vi "deceltobun.vi"() -> ()   [LabVIEW 2014, in "Panels.lvlib"]
uses:
  Panels.lvlib
  CSlibraries-extern/DimLVEvent/DimIndicators/DimIndicators.lvlib
  CSlibraries/UtilityLib/UtilityLib.lvlib
  CS_Core/CSSystem/CoreLib/CoreLib.lvlib
  CSlibraries/UtilityLib/UtilityLib.valueStatus.ctl
  CSlibraries-extern/DimLVEvent/LVDimInterface/LVDimInterface.lvlib
  Instance           1 18Saved   deceltobun .vi
  Instance           2 18Saved   deceltobun .vi
  CSlibraries-extern/DimLVEvent/DimIndicators/DimIndicators.numericArrayType.ctl
  CSlibraries-extern/DimLVEvent/DimIndicators/DimIndicators.anyType.ctl
  CSlibraries-extern/DimLVEvent/DimIndicators/DimIndicators.numericType.ctl
panel:
  out "DIM Error":bool
  in  "SetFileLocation_Data":T1={"data"="NOLINK", "no link"=TRUE, "quality"=-1, "timeStamp"=0.0}
  in  "Q90PlanDefY":bool
  in  "ISDefY":bool
  in  "Q90PlanLens":bool
  in  "BOB3DefY":bool
  in  "BOB3DefX":bool
  in  "BOB2Q90Lens":bool
  in  "Q90DefMain":bool
  in  "Q90BOB3Lens":bool
  in  "ISDefX":bool
  in  "Q90CylLens":bool
  in  "BOB2DefX":bool
  in  "BOB2DefY":bool
  in  "DecelLens":bool
  in  "Decel":bool
  in  "PreBunLens":bool
  in  "Q90DefMain_MonData":T2={"data"=inf, "no link"=FALSE, "quality"=1, "timeStamp"=3265900746.554}
  in  "Q90BOB3Lens_MonData":T2={"data"=inf, "no link"=FALSE, "quality"=1, "timeStamp"=3265900746.538}
  in  "Q90PlanLens_MonData":T2={"data"=inf, "no link"=FALSE, "quality"=1, "timeStamp"=3265900746.522}
  in  "BOB3DefX_MonData":T2={"data"=inf, "no link"=FALSE, "quality"=1, "timeStamp"=3265900746.554}
  in  "Decel_MonData":T2={"data"=inf, "no link"=FALSE, "quality"=1, "timeStamp"=3265900746.538}
  in  "DecelLens_MonData":T2={"data"=inf, "no link"=FALSE, "quality"=1, "timeStamp"=3265900746.569}
  in  "BOB2Q90Lens_MonData":T2={"data"=inf, "no link"=FALSE, "quality"=1, "timeStamp"=3265900746.554}
  in  "ISDefX_MonData":T2={"data"=inf, "no link"=FALSE, "quality"=1, "timeStamp"=3265900746.538}
  in  "BOB2DefX_MonData":T2={"data"=inf, "no link"=FALSE, "quality"=1, "timeStamp"=3265900746.569}
  in  "BOB3DefY_MonData":T2={"data"=inf, "no link"=FALSE, "quality"=1, "timeStamp"=3265900746.569}
  in  "Q90DefCorr1_MonData":T2={"data"=inf, "no link"=FALSE, "quality"=1, "timeStamp"=3265900746.538}
  in  "Q90DefCorr2_MonData":T2={"data"=inf, "no link"=FALSE, "quality"=1, "timeStamp"=3265900746.585}
  in  "Q90PlanDefY_MonData":T2={"data"=inf, "no link"=FALSE, "quality"=1, "timeStamp"=3265900746.538}
  in  "Q90DefMain1_MonData":T2={"data"=inf, "no link"=FALSE, "quality"=1, "timeStamp"=3265900746.554}
  in  "ISDefY_MonData":T2={"data"=inf, "no link"=FALSE, "quality"=1, "timeStamp"=3265900746.522}
  in  "PreBunLens_MonData":T2={"data"=inf, "no link"=FALSE, "quality"=1, "timeStamp"=3265900746.538}
  in  "BOB2DefY_MonData":T2={"data"=inf, "no link"=FALSE, "quality"=1, "timeStamp"=3265900746.6}
  in  "Q90CylLens_MonData":T2={"data"=inf, "no link"=FALSE, "quality"=1, "timeStamp"=3265900746.585}
  in  "Q90DefMain2_MonData":T2={"data"=inf, "no link"=FALSE, "quality"=1, "timeStamp"=3265900746.569}
  in  "Q90DefMain_SetValueInfoData":T3={"data"=[-400.0, 400.0, 3.0], "no link"=FALSE, "quality"=0, "timeStamp"=3265900746.554}
  in  "Q90DefMain_SetData":T3={"data"=[0.0, 0.0, 0.0, 0.0], "no link"=FALSE, "quality"=1, "timeStamp"=3265900745.1}
  out "Q90DefMain_Mon":dbl=inf format="%.4f"
  in  "Decel_SetValueInfoData":T3={"data"=[-404.0, 401.8, 3.0], "no link"=FALSE, "quality"=0, "timeStamp"=3265900746.569}
  in  "Decel_SetData":T3={"data"=[0.0, 0.0, 0.0, 0.0], "no link"=FALSE, "quality"=1, "timeStamp"=3265900745.053}
  out "BOB3DefX_Mon":dbl=inf format="%.4f"
  in  "PreBunLens_SetData":T3={"data"=[0.0, 0.0, 0.0, 0.0], "no link"=FALSE, "quality"=1, "timeStamp"=3265900745.053}
  in  "BOB3DefY_SetValueInfoData":T3={"data"=[-400.0, 400.0, 3.0], "no link"=FALSE, "quality"=0, "timeStamp"=3265900746.554}
  in  "BOB3DefX_SetValueInfoData":T3={"data"=[-400.0, 400.0, 3.0], "no link"=FALSE, "quality"=0, "timeStamp"=3265900746.538}
  in  "Q90BOB3Lens_SetValueInfoData":T3={"data"=[-400.0, 400.0, 3.0], "no link"=FALSE, "quality"=0, "timeStamp"=3265900746.522}
  in  "ISDefY_SetValueInfoData":T3={"data"=[-118.7, 118.8, 3.0], "no link"=FALSE, "quality"=0, "timeStamp"=3265900746.569}
  in  "Q90PlanDefY_SetValueInfoData":T3={"data"=[-120.9, 120.5, 3.0], "no link"=FALSE, "quality"=0, "timeStamp"=3265900746.585}
  in  "Q90PlanLens_SetValueInfoData":T3={"data"=[-120.8, 120.3, 3.0], "no link"=FALSE, "quality"=0, "timeStamp"=3265900746.569}
  in  "BOB3DefY_SetData":T3={"data"=[0.0, 0.0, 0.0, 0.0], "no link"=FALSE, "quality"=1, "timeStamp"=3265900745.1}
  in  "BOB3DefX_SetData":T3={"data"=[0.0, 0.0, 0.0, 0.0], "no link"=FALSE, "quality"=1, "timeStamp"=3265900745.085}
  in  "Q90BOB3Lens_SetData":T3={"data"=[0.0, 0.0, 0.0, 0.0], "no link"=FALSE, "quality"=1, "timeStamp"=3265900745.069}
  in  "ISDefY_SetData":T3={"data"=[0.0, 0.0, 0.0, 0.0], "no link"=FALSE, "quality"=1, "timeStamp"=3265900745.069}
  in  "Q90PlanDefY_SetData":T3={"data"=[0.0, 0.0, 0.0, 0.0], "no link"=FALSE, "quality"=1, "timeStamp"=3265900745.069}
  out "Q90PlanLens_Mon":dbl=inf format="%.4f"
  out "Q90BOB3Lens_Mon":dbl=inf format="%.4f"
  out "BOB3DefY_Mon":dbl=inf format="%.4f"
  out "Q90DefMain1_Mon":dbl=inf format="%.4f"
  out "Q90DefCorr2_Mon":dbl=inf format="%.4f"
  out "Q90DefCorr1_Mon":dbl=inf format="%.4f"
  out "Q90PlanDefY_Mon":dbl=inf format="%.4f"
  in  "Q90PlanLens_SetData":T3={"data"=[0.0, 0.0, 0.0, 0.0], "no link"=FALSE, "quality"=1, "timeStamp"=3265900745.069}
  out "DecelLens_Mon":dbl=inf format="%.4f"
  out "Decel_Mon":dbl=inf format="%.4f"
  out "i ref out":refnum<vi>
  in  "Last Loaded File_Data":T1={"data"="NOLINK", "no link"=TRUE, "quality"=-1, "timeStamp"=0.0}
  out "FileUpToDate":bool=TRUE caption="Parameter Changed"
  in  "Close All Panels":bool
  in  "DecelLens_SetValueInfoData":T3={"data"=[-401.3, 400.4, 3.0], "no link"=FALSE, "quality"=0, "timeStamp"=3265900746.554}
  in  "BOB2Q90Lens_SetValueInfoData":T3={"data"=[-404.3, 403.0, 3.0], "no link"=FALSE, "quality"=0, "timeStamp"=3265900746.538}
  in  "BOB2DefX_SetValueInfoData":T3={"data"=[-400.3, 399.3, 3.0], "no link"=FALSE, "quality"=0, "timeStamp"=3265900746.569}
  in  "BOB2DefY_SetValueInfoData":T3={"data"=[0.0, 3000.0, -1.0], "no link"=FALSE, "quality"=0, "timeStamp"=3265900746.554}
  in  "Q90CylLens_SetValueInfoData":T3={"data"=[0.0, 1500.0, -1.0], "no link"=FALSE, "quality"=0, "timeStamp"=3265900746.554}
  in  "ISDefX_SetValueInfoData":T3={"data"=[0.0, 1000.0, -1.0], "no link"=FALSE, "quality"=0, "timeStamp"=3265900746.538}
  in  "PreBunLens_SetValueInfoData":T3={"data"=[-404.0, 401.8, 3.0], "no link"=FALSE, "quality"=0, "timeStamp"=3265900746.569}
  in  "ISDefX_SetData":T3={"data"=[0.0, 0.0, 0.0, 0.0], "no link"=FALSE, "quality"=1, "timeStamp"=3265900745.069}
  in  "Q90CylLens_SetData":T3={"data"=[0.0, 0.0, 0.0, 0.0], "no link"=FALSE, "quality"=1, "timeStamp"=3265900745.053}
  in  "BOB2DefY_SetData":T3={"data"=[0.0, 0.0, 0.0, 0.0], "no link"=FALSE, "quality"=1, "timeStamp"=3265900745.085}
  in  "BOB2DefX_SetData":T3={"data"=[0.0, 0.0, 0.0, 0.0], "no link"=FALSE, "quality"=1, "timeStamp"=3265900745.085}
  in  "BOB2Q90Lens_SetData":T3={"data"=[0.0, 0.0, 0.0, 0.0], "no link"=FALSE, "quality"=1, "timeStamp"=3265900745.085}
  in  "DecelLens_SetData":T3={"data"=[0.0, 0.0, 0.0, 0.0], "no link"=FALSE, "quality"=1, "timeStamp"=3265900745.053}
  out "Last Loaded File":string
  in  "SetFileLocation":path=path "\\\\Projects\\proj1/lebit/Data Exchange/data/bob1tobunControl"
  out "ISDefY_Mon":dbl=inf format="%.4f"
  out "Q90CylLens_Mon":dbl=inf format="%.4f"
  out "PreBunLens_Mon":dbl=inf format="%.4f"
  out "BOB2DefY_Mon":dbl=inf format="%.4f"
  out "Q90DefMain2_Mon":dbl=inf format="%.4f"
  out "BOB2DefX_Mon":dbl=inf format="%.4f"
  out "ISDefX_Mon":dbl=inf format="%.4f"
  out "BOB2Q90Lens_Mon":dbl=inf format="%.4f"
  # "Parameter changed, data file is no longer up-to-date."
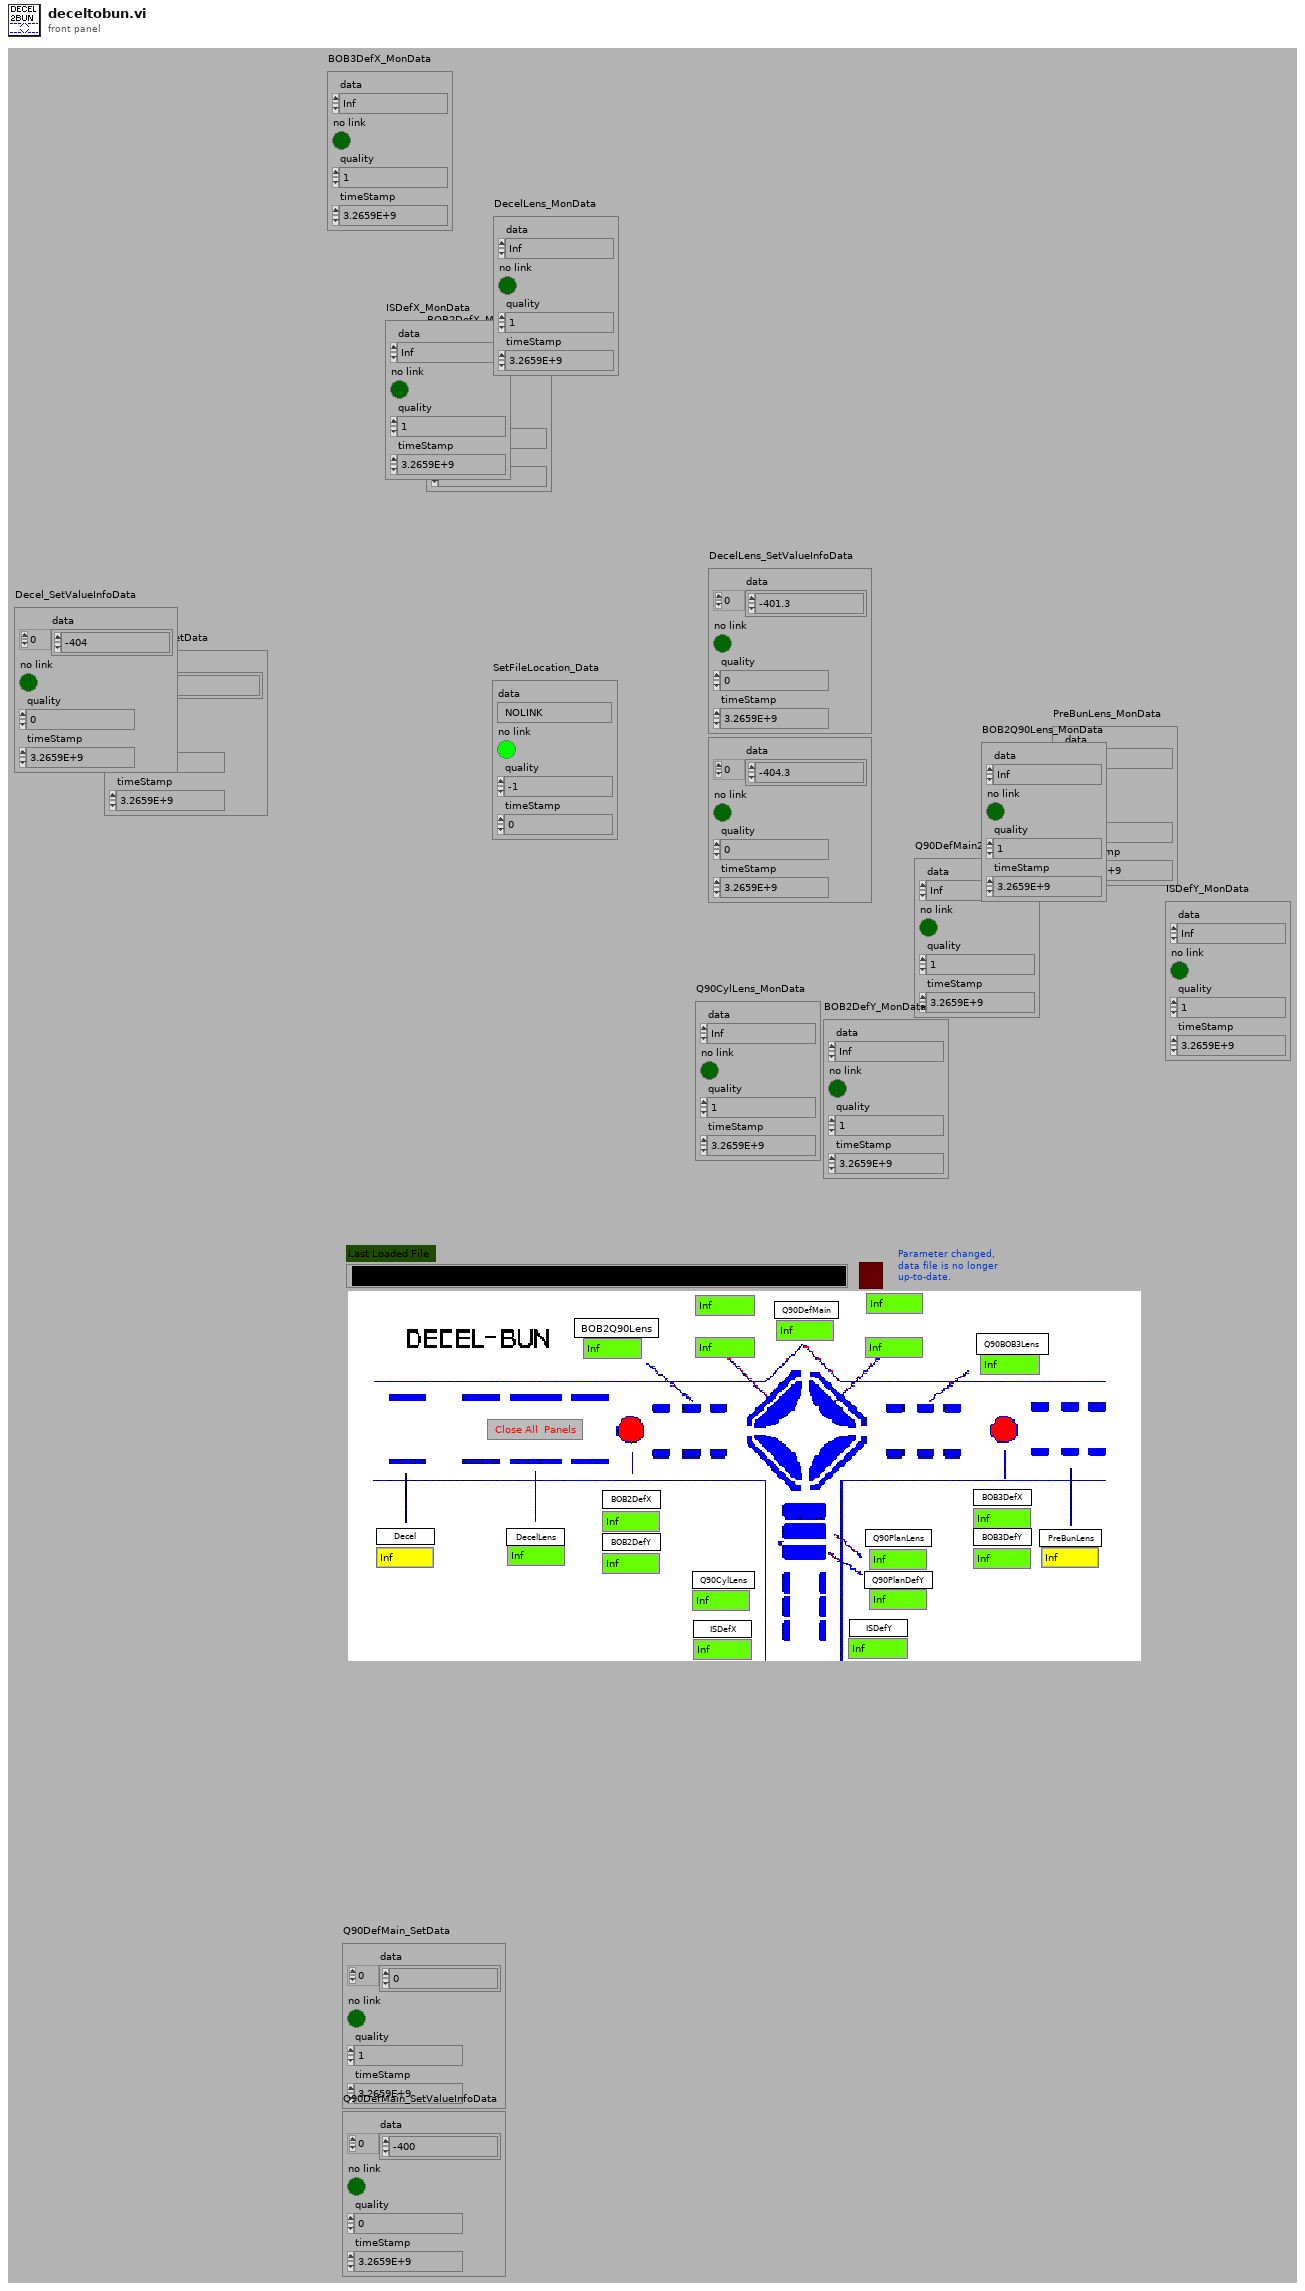
[diagram p1: front panel]
types:
  T1 = typedef "DimIndicators.lvlib/DimIndicators.anyType.ctl" = cluster{"data":string, "no link":bool, "quality":i32, "timeStamp":dbl}
  T2 = typedef "DimIndicators.lvlib/DimIndicators.numericType.ctl" = cluster{"data":dbl, "no link":bool, "quality":i32, "timeStamp":dbl}
  T3 = typedef "DimIndicators.lvlib/DimIndicators.numericArrayType.ctl" = cluster{"data":dbl[], "no link":bool, "quality":i32, "timeStamp":dbl}
  T4 = typedef "UtilityLib.lvlib/UtilityLib.valueStatus.ctl" = enum16{"no info available", "stand by/off", "on", "warning", "alarm/malfunction", "not implemented", "user action required", "important information", "system default", "control default", "indicator default", "button default"}
  T5 = cluster{"data":string, "no link":bool, "quality":i32, "timeStamp":dbl}
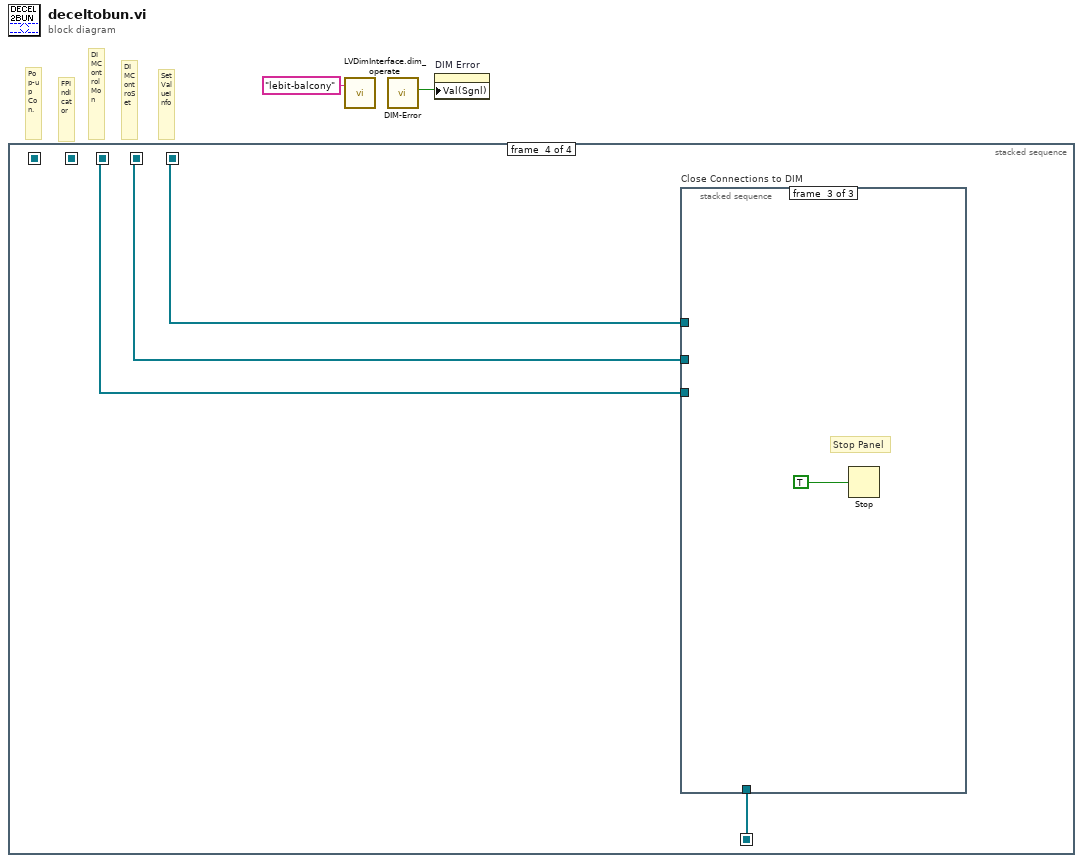
[diagram p0: block diagram]
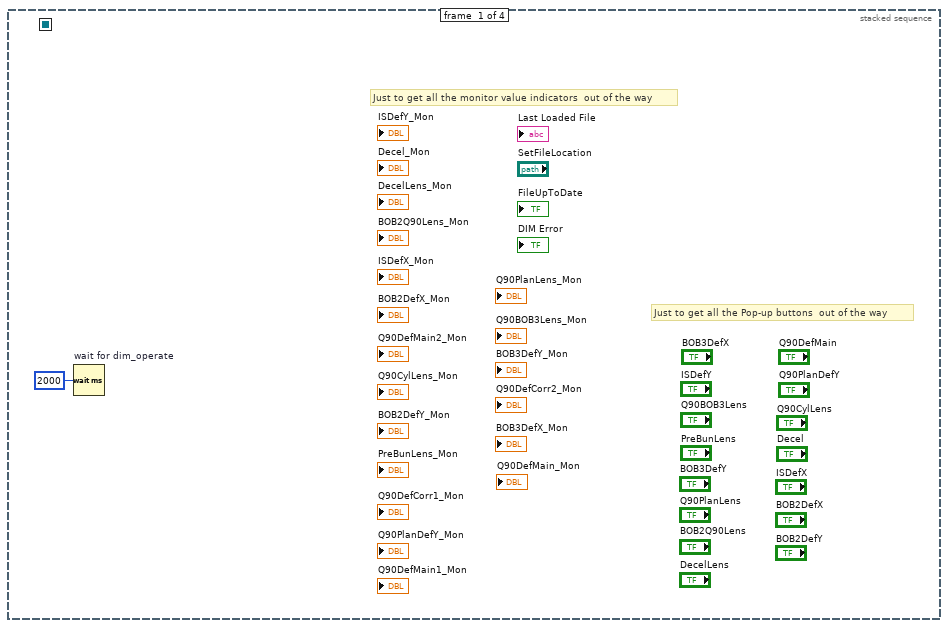
[diagram p2: hidden frame]
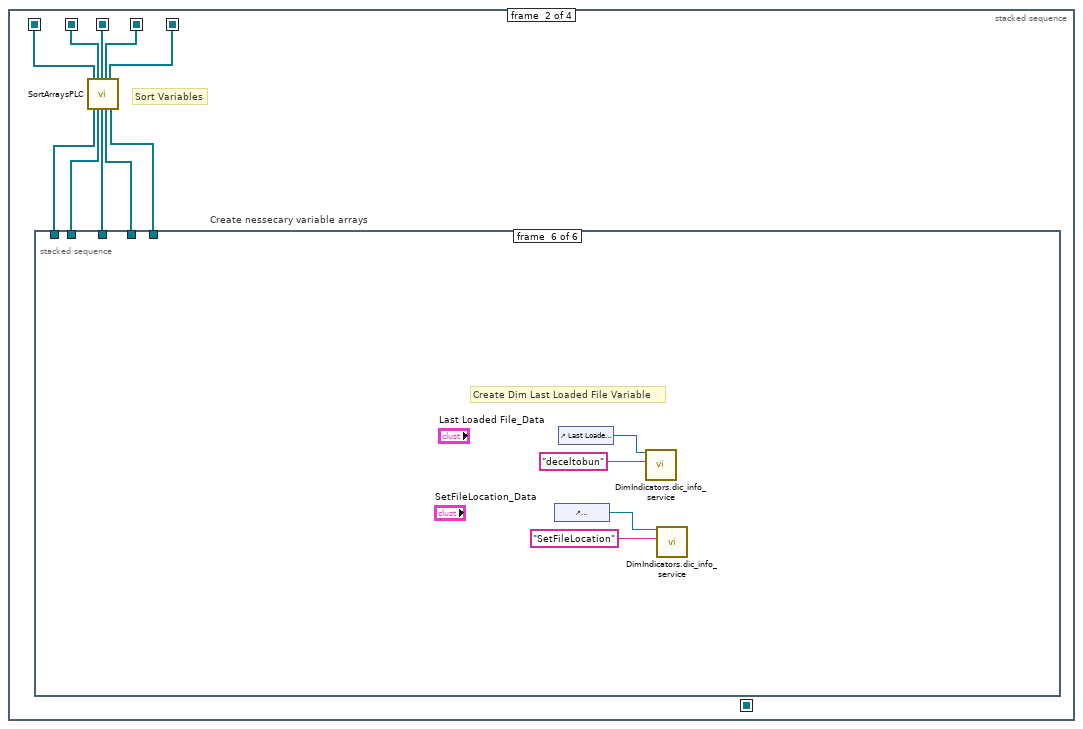
[diagram p3: hidden frame]
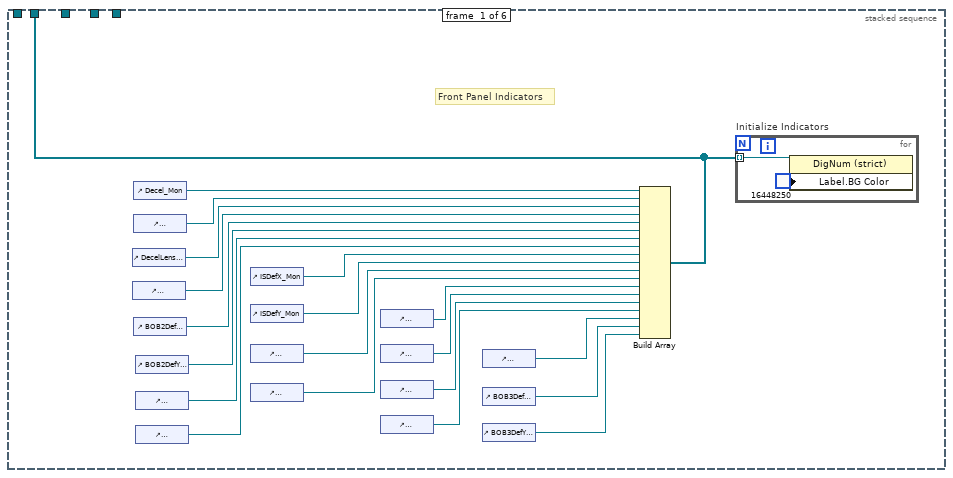
[diagram p4: hidden frame]
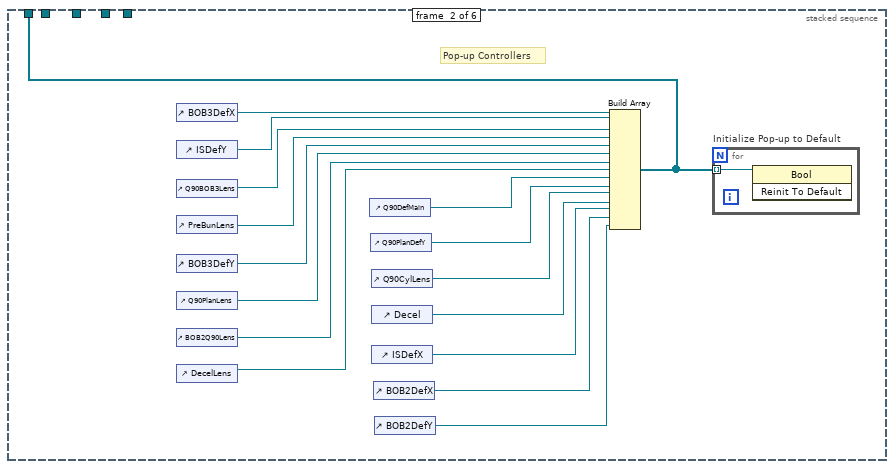
[diagram p5: hidden frame]
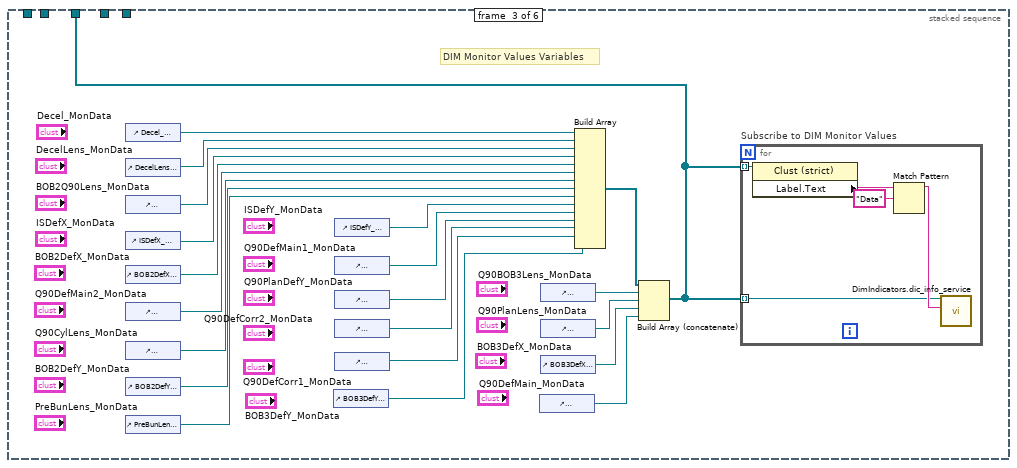
[diagram p6: hidden frame]
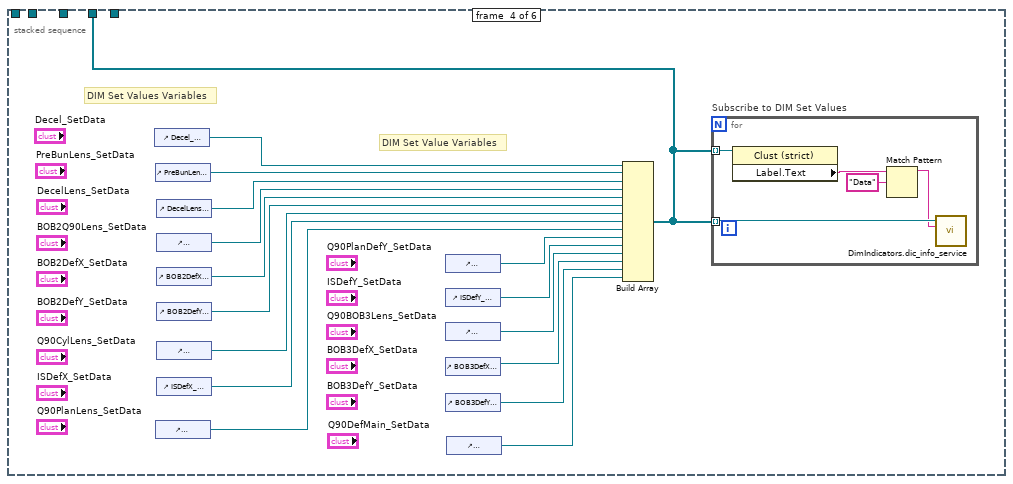
[diagram p7: hidden frame]
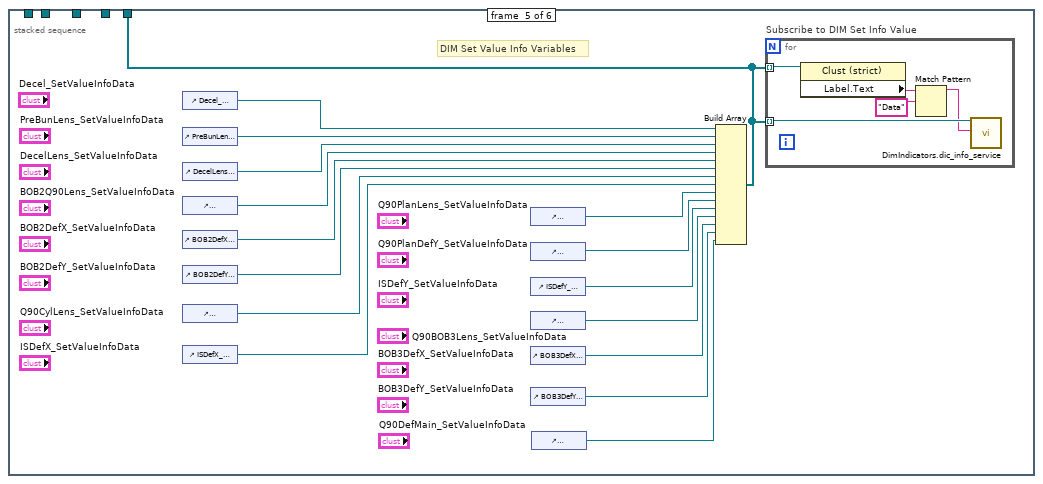
[diagram p8: hidden frame]
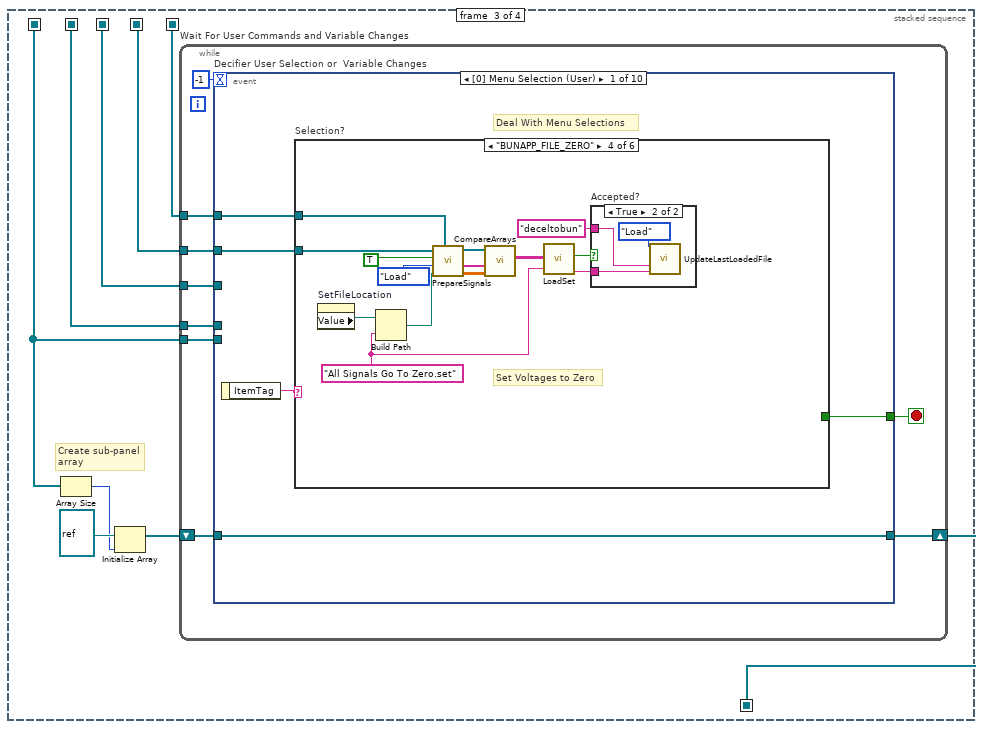
[diagram p9: hidden frame]
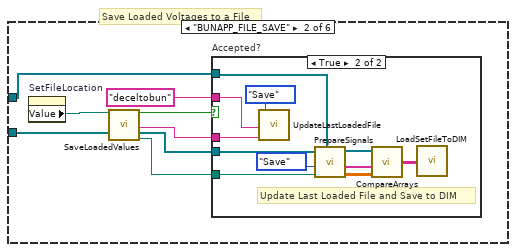
[diagram p11: hidden frame]
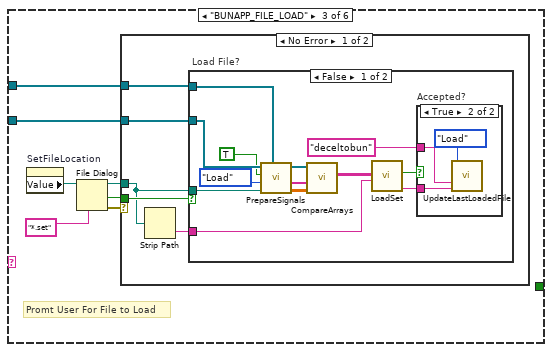
[diagram p13: hidden frame]
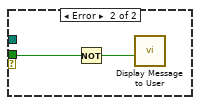
[diagram p16: hidden frame]
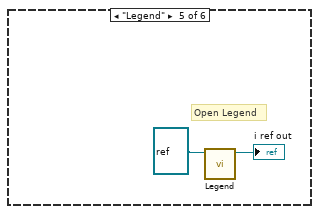
[diagram p18: hidden frame]
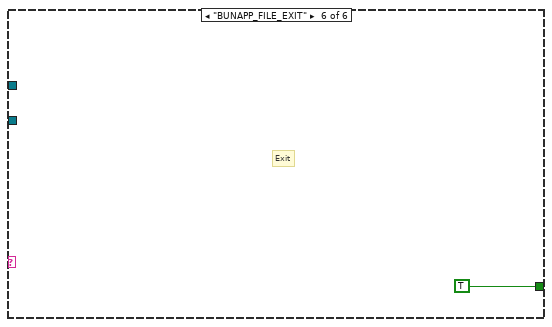
[diagram p19: hidden frame]
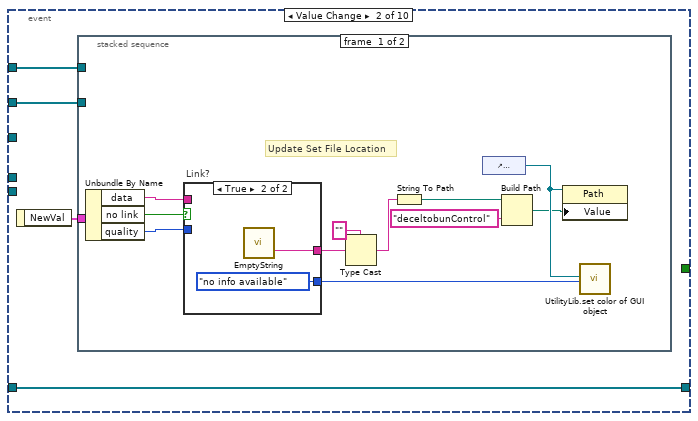
[diagram p20: hidden frame]
diagram:
  # "Pop-up Con."
  # "SetValueInfo"
  # "DIMControSet"
  # "DIMControlMon"
  # "FPIndicator"
  n1 = stacked-sequence {
    seq-local: [_ w5 _ _] -> [_ _ w131 _]
    seq-local: [_ w6 _ _] -> [_ _ w126 w328]
    seq-local: [_ _ w129 _] -> [_ _ _ w327]
    seq-local: [_ w7 _ _] -> [_ _ w128 w326]
    seq-local: [_ w8 _ _] -> [_ _ w127 w325]
    seq-local: [_ w4 _ _] -> [_ _ w125 _]
    frame #0 {
      # "Just to get all the Pop-up buttons  out of the way"
      # "Just to get all the monitor value indicators  out of the way"
      n2 = Wait (ms) "wait for dim_operate"(milliseconds to wait=u32 2000) -> ()  [unwired: 1 out]
    }
    frame #1 {
      # "Sort Variables"
      # "Arrange references to all monitor-value related buttons into an array."
      n3 = stacked-sequence "Create nessecary variable arrays" {
        tunnel: [w32 _ _ _ _ _] -> w12
        tunnel: [_ w36 _ _ _ _] -> w13
        tunnel: [_ _ w53 _ _ _] -> w11
        tunnel: [_ _ _ w79 _ _] -> w10
        tunnel: [_ _ _ _ w100 _] -> w9
        frame #0 {
          # "Front Panel Indicators"
          n4 = control-ref of="DecelLens_Mon"() -> (w25:refnum<vi>)
          n5 = control-ref of="BOB2Q90Lens_Mon"() -> (w24:refnum<vi>)
          n6 = control-ref of="Decel_Mon"() -> (w31:refnum<vi>)
          n7 = control-ref of="PreBunLens_Mon"() -> (w26:refnum<vi>)
          n8 = control-ref of="BOB2DefX_Mon"() -> (w33:refnum<vi>)
          n9 = control-ref of="BOB2DefY_Mon"() -> (w22:refnum<vi>)
          n10 = control-ref of="Q90DefMain2_Mon"() -> (w21:refnum<vi>)
          n11 = control-ref of="Q90CylLens_Mon"() -> (w20:refnum<vi>)
          n12 = control-ref of="ISDefX_Mon"() -> (w23:refnum<vi>)
          n13 = control-ref of="ISDefY_Mon"() -> (w30:refnum<vi>)
          n14 = control-ref of="Q90DefMain_Mon"() -> (w18:refnum<vi>)
          n15 = control-ref of="Q90DefMain1_Mon"() -> (w17:refnum<vi>)
          n16 = control-ref of="Q90DefCorr2_Mon"() -> (w29:refnum<vi>)
          n17 = control-ref of="Q90DefCorr1_Mon"() -> (w28:refnum<vi>)
          n18 = control-ref of="Q90PlanLens_Mon"() -> (w16:refnum<vi>)
          n19 = control-ref of="Q90PlanDefY_Mon"() -> (w15:refnum<vi>)
          n20 = control-ref of="Q90BOB3Lens_Mon"() -> (w14:refnum<vi>)
          n21 = control-ref of="BOB3DefX_Mon"() -> (w27:refnum<vi>)
          n22 = control-ref of="BOB3DefY_Mon"() -> (w19:refnum<vi>)
          n23 = Build Array(w31, w26, w25, w24, w33, w22, w21, w20, w23, w30, w18, w17, w29, w28, w16, w15, w14, w27, w19) -> (w32:refnum<vi>[])
          n24 = for "Initialize Indicators" {
            tunnel: w32 -> [w35] mode=indexing
            n25 = property class="DigNum (strict)"(reference=w35, "Label.BG Color"=u32 16448250 ("Color Box")) -> ()  [unwired: 1 in, 2 out]
          }
        }
        frame #1 {
          # "Pop-up Controllers"
          n26 = control-ref of="BOB3DefX"() -> (w51:refnum<vi>)
          n27 = control-ref of="ISDefY"() -> (w50:refnum<vi>)
          n28 = control-ref of="Q90BOB3Lens"() -> (w49:refnum<vi>)
          n29 = control-ref of="PreBunLens"() -> (w48:refnum<vi>)
          n30 = control-ref of="BOB3DefY"() -> (w47:refnum<vi>)
          n31 = control-ref of="Q90PlanLens"() -> (w46:refnum<vi>)
          n32 = control-ref of="BOB2Q90Lens"() -> (w45:refnum<vi>)
          n33 = control-ref of="DecelLens"() -> (w44:refnum<vi>)
          n34 = control-ref of="Q90DefMain"() -> (w43:refnum<vi>)
          n35 = control-ref of="Q90PlanDefY"() -> (w42:refnum<vi>)
          n36 = control-ref of="Q90CylLens"() -> (w41:refnum<vi>)
          n37 = control-ref of="Decel"() -> (w40:refnum<vi>)
          n38 = control-ref of="ISDefX"() -> (w39:refnum<vi>)
          n39 = control-ref of="BOB2DefX"() -> (w38:refnum<vi>)
          n40 = control-ref of="BOB2DefY"() -> (w37:refnum<vi>)
          n41 = Build Array(w51, w50, w49, w48, w47, w46, w45, w44, w43, w42, w41, w40, w39, w38, w37) -> (w36:refnum<vi>[])
          n42 = for "Initialize Pop-up to Default" {
            tunnel: w36 -> [w52] mode=indexing
            n43 = invoke class="Bool" method="Reinit To Default"(reference=w52) -> ()  [unwired: 2 in, 3 out]
          }
        }
        frame #2 {
          # "DIM Monitor Values Variables"
          n44 = control-ref of="Decel_MonData"() -> (w69:refnum<vi>)
          n45 = control-ref of="DecelLens_MonData"() -> (w68:refnum<vi>)
          n46 = control-ref of="BOB2Q90Lens_MonData"() -> (w67:refnum<vi>)
          n47 = control-ref of="ISDefX_MonData"() -> (w62:refnum<vi>)
          n48 = control-ref of="BOB2DefX_MonData"() -> (w63:refnum<vi>)
          n49 = control-ref of="Q90DefMain2_MonData"() -> (w55:refnum<vi>)
          n50 = control-ref of="Q90CylLens_MonData"() -> (w56:refnum<vi>)
          n51 = control-ref of="BOB2DefY_MonData"() -> (w57:refnum<vi>)
          n52 = control-ref of="PreBunLens_MonData"() -> (w58:refnum<vi>)
          n53 = control-ref of="BOB3DefY_MonData"() -> (w54:refnum<vi>)
          n54 = control-ref of="ISDefY_MonData"() -> (w59:refnum<vi>)
          n55 = control-ref of="Q90DefMain1_MonData"() -> (w60:refnum<vi>)
          n56 = control-ref of="Q90PlanDefY_MonData"() -> (w61:refnum<vi>)
          n57 = control-ref of="Q90DefCorr2_MonData"() -> (w70:refnum<vi>)
          n58 = control-ref of="Q90DefCorr1_MonData"() -> (w71:refnum<vi>)
          n59 = control-ref of="Q90DefMain_MonData"() -> (w73:refnum<vi>)
          n60 = control-ref of="Q90BOB3Lens_MonData"() -> (w64:refnum<vi>)
          n61 = control-ref of="Q90PlanLens_MonData"() -> (w65:refnum<vi>)
          n62 = control-ref of="BOB3DefX_MonData"() -> (w66:refnum<vi>)
          n63 = Build Array(w69, w68, w67, w62, w63, w55, w56, w57, w58, w59, w60, w61, w70, w71, w54) -> (w72:refnum<vi>[])
          n64 = Build Array (concatenate)(w72, w64, w65, w66, w73) -> (w53:refnum<vi>[])
          n65 = for "Subscribe to DIM Monitor Values" {
            tunnel: w53 -> [w75] mode=indexing
            tunnel: w53 -> [w74] mode=indexing
            n66 = property class="Clust (strict)"(reference=w74) -> ("Label.Text"=w77:string)  [unwired: 1 in, 2 out]
            n67 = Match Pattern(string=w77, regular expression="Data") -> (before substring=w76:string)  [unwired: 1 in, 3 out]
            n68 = call "DimIndicators.dic_info_service.vi"("controlRef"=w75, "serviceName"=w76) -> ()  [unwired: 16 in, 2 out]
          }
        }
        frame #3 {
          # "DIM Set Value Variables"
          # "DIM Set Values Variables"
          n69 = control-ref of="Decel_SetData"() -> (w81:refnum<vi>)
          n70 = control-ref of="PreBunLens_SetData"() -> (w82:refnum<vi>)
          n71 = control-ref of="Q90PlanLens_SetData"() -> (w88:refnum<vi>)
          n72 = control-ref of="DecelLens_SetData"() -> (w94:refnum<vi>)
          n73 = control-ref of="BOB2Q90Lens_SetData"() -> (w93:refnum<vi>)
          n74 = control-ref of="BOB2DefX_SetData"() -> (w92:refnum<vi>)
          n75 = control-ref of="BOB2DefY_SetData"() -> (w91:refnum<vi>)
          n76 = control-ref of="Q90CylLens_SetData"() -> (w90:refnum<vi>)
          n77 = control-ref of="ISDefX_SetData"() -> (w89:refnum<vi>)
          n78 = control-ref of="Q90PlanDefY_SetData"() -> (w87:refnum<vi>)
          n79 = control-ref of="ISDefY_SetData"() -> (w86:refnum<vi>)
          n80 = control-ref of="Q90BOB3Lens_SetData"() -> (w85:refnum<vi>)
          n81 = control-ref of="BOB3DefX_SetData"() -> (w84:refnum<vi>)
          n82 = control-ref of="BOB3DefY_SetData"() -> (w83:refnum<vi>)
          n83 = control-ref of="Q90DefMain_SetData"() -> (w80:refnum<vi>)
          n84 = Build Array(w81, w82, w94, w93, w92, w91, w90, w89, w88, w87, w86, w85, w84, w83, w80) -> (w79:refnum<vi>[])
          n85 = for "Subscribe to DIM Set Values" {
            tunnel: w79 -> [w95] mode=indexing
            tunnel: w79 -> [w99] mode=indexing
            n86 = property class="Clust (strict)"(reference=w95) -> ("Label.Text"=w98:string)  [unwired: 1 in, 2 out]
            n87 = Match Pattern(string=w98, regular expression="Data") -> (before substring=w96:string)  [unwired: 1 in, 3 out]
            n88 = call "DimIndicators.dic_info_service.vi"("controlRef"=w99, "serviceName"=w96) -> ()  [unwired: 16 in, 2 out]
          }
        }
        frame #4 {
          # "DIM Set Value Info Variables"
          n89 = control-ref of="Decel_SetValueInfoData"() -> (w102:refnum<vi>)
          n90 = control-ref of="PreBunLens_SetValueInfoData"() -> (w115:refnum<vi>)
          n91 = control-ref of="DecelLens_SetValueInfoData"() -> (w114:refnum<vi>)
          n92 = control-ref of="BOB2Q90Lens_SetValueInfoData"() -> (w113:refnum<vi>)
          n93 = control-ref of="BOB2DefX_SetValueInfoData"() -> (w112:refnum<vi>)
          n94 = control-ref of="BOB2DefY_SetValueInfoData"() -> (w111:refnum<vi>)
          n95 = control-ref of="Q90CylLens_SetValueInfoData"() -> (w110:refnum<vi>)
          n96 = control-ref of="ISDefX_SetValueInfoData"() -> (w109:refnum<vi>)
          n97 = control-ref of="Q90PlanLens_SetValueInfoData"() -> (w108:refnum<vi>)
          n98 = control-ref of="Q90PlanDefY_SetValueInfoData"() -> (w107:refnum<vi>)
          n99 = control-ref of="ISDefY_SetValueInfoData"() -> (w106:refnum<vi>)
          n100 = control-ref of="Q90BOB3Lens_SetValueInfoData"() -> (w105:refnum<vi>)
          n101 = control-ref of="BOB3DefX_SetValueInfoData"() -> (w104:refnum<vi>)
          n102 = control-ref of="BOB3DefY_SetValueInfoData"() -> (w103:refnum<vi>)
          n103 = control-ref of="Q90DefMain_SetValueInfoData"() -> (w101:refnum<vi>)
          n104 = Build Array(w102, w115, w114, w113, w112, w111, w110, w109, w108, w107, w106, w105, w104, w103, w101) -> (w100:refnum<vi>[])
          n105 = for "Subscribe to DIM Set Info Value" {
            tunnel: w100 -> [w116] mode=indexing
            tunnel: w100 -> [w120] mode=indexing
            n106 = property class="Clust (strict)"(reference=w116) -> ("Label.Text"=w119:string)  [unwired: 1 in, 2 out]
            n107 = Match Pattern(string=w119, regular expression="Data") -> (before substring=w117:string)  [unwired: 1 in, 3 out]
            n108 = call "DimIndicators.dic_info_service.vi"("controlRef"=w120, "serviceName"=w117) -> ()  [unwired: 16 in, 2 out]
          }
        }
        frame #5 {
          # "Create Dim Last Loaded File Variable"
          n109 = control-ref of="SetFileLocation_Data"() -> (w124:refnum<vi>)
          n110 = control-ref of="Last Loaded File_Data"() -> (w122:refnum<vi>)
          n111 = call "DimIndicators.dic_info_service.vi"("controlRef"=w122, "serviceName"="deceltobun" ("string")) -> ()  [unwired: 16 in, 2 out]
          n112 = call "DimIndicators.dic_info_service.vi"("controlRef"=w124, "serviceName"="SetFileLocation" ("string")) -> ()  [unwired: 16 in, 2 out]
        }
      }
      n113 = call "SortArraysPLC.vi"("Pop-up Con."=w13, "FPIndicator in"=w12, "DIMControlMon"=w11, "DIMControSet"=w10, "SetValueInfo"=w9) -> ("Pop-up Con. out"=w4:refnum<vi>[], "FPIndicator out"=w5:refnum<vi>[], "DIMControlMon out"=w6:refnum<vi>[], "DIMControSet out"=w7:refnum<vi>[], "SetValueInfo out"=w8:refnum<vi>[])  [unwired: 18 in]
    }
    frame #2 {
      # "Create sub-panel\narray"
      n114 = Array Size(array=w125) -> (size(s)=w130:i32)
      n115 = Initialize Array(refnum<vi> refnum ("vi reference"), w130) -> (w133:refnum<vi>[])
      n116 = while "Wait For User Commands and Variable Changes" {
        tunnel: w131 -> [w142]
        shift-right: [w140] -> w129
        shift-left: w133 -> [w141]
        tunnel: w128 -> [w139]
        tunnel: w127 -> [w138]
        tunnel: w126 -> [w136]
        tunnel: w125 -> [w135]
        stop <- w134 stop-if-true
        n117 = event "Decifier User Selection or  Variable Changes" shown="[0] Menu Selection (User)" {
          selector: _ -> [_ _ _ _ _ _ _ _ _ _]
          dyn-events: _ -> [_ _ _ _ _ _ _ _ _ _]
          timeout: -1 -> [_ _ _ _ _ _ _ _ _ _]
          tunnel: [w144 _ _ _ _ _ _ w297 _ TRUE ("stop")] -> w134
          tunnel: w142 -> [_ _ _ w254 _ _ _ _ _ _]
          tunnel: w141 -> [w147 w219 w251 w258 w276 w284 w291 w298 w299 w303]
          tunnel: [w147 w219 w251 w258 w276 w282 w289 w298 w299 _] -> w140
          tunnel: w139 -> [w145 w218 w246 _ w274 _ _ _ _ w301]
          tunnel: w138 -> [w143 w217 w245 _ _ _ _ _ _ w302]
          tunnel: w136 -> [_ _ _ w257 _ _ _ _ _ w300]
          tunnel: w135 -> [_ _ _ _ _ w277 _ _ _ _]
          event Menu Selection (User) {
            # "Deal With Menu Selections"
            n118 = event-data() -> ("ItemTag"=w146:string)  [unwired: 1 in]
            n119 = case "Selection?" shown="\"BUNAPP_FILE_ZERO\"" w146 {
              tunnel: w145 -> [_ w152 w172 w210 _ _]
              tunnel: [_ _ _ _ _ TRUE ("stop")] -> w144
              tunnel: w143 -> [_ w148 w167 w197 _ _]
              frame "False", Default {
              }
              frame "BUNAPP_FILE_SAVE" {
                # "Save Loaded Voltages to a File"
                n120 = property on="SetFileLocation" class="Path"() -> ("Value"=w153:path)  [unwired: 2 in, 2 out]
                n121 = call "SaveLoadedValues.vi"("Panel Location?"=w153, "DIMControlSet in"=w152) -> ("File Saved?"=w154:bool, "File Name"=w151:string, "DIMControlSet out"=w149:refnum<vi>[], "Path"=w150:path)  [unwired: 14 in]
                n122 = case "Accepted?" shown="True" w154 {
                  tunnel: w151 -> [_ w164]
                  tunnel: "deceltobun" ("string") -> [_ w166]
                  tunnel: w149 -> [_ w165]
                  tunnel: w150 -> [_ w163]
                  tunnel: w148 -> [_ w157]
                  frame False {
                  }
                  frame True {
                    # "Update Last Loaded File and Save to DIM"
                    n123 = call "UpdateLastLoadedFile.vi"("LoadOrSave"=enum16{"Load", "Save"}."Save", "GUIName"=w166, "FileNameIn"=w164) -> ()  [unwired: 13 in]
                    n124 = call "PrepareSignals.vi"("SetValueInfo in"=w157, "setfile path"=w163, "Enum"=enum16{"Save", "Load"}."Save", "DIMControSet in"=w165) -> ("indexed loaded Array"=w161:dbl[][], "Name Array"=w162:string[], "DIMControSet out"=w160:refnum<vi>[])  [unwired: 5 in]
                    n125 = call "CompareArrays.vi"("indexed loaded Array"=w161, "Name Array"=w162, "DIMControSet"=w160) -> ("Table for loading values"=w159:string[][])  [unwired: 4 in]
                    n126 = call "LoadSetFileToDIM.vi"("output array"=w159) -> ()  [unwired: 2 in]
                  }
                }
              }
              frame "BUNAPP_FILE_LOAD" {
                # "Promt User For File to Load"
                n127 = property on="SetFileLocation" class="Path"() -> ("Value"=w169:path)  [unwired: 2 in, 2 out]
                n128 = File Dialog(6:"*.set" ("pattern (all files)"), 11:w169) -> (0:w168:errorcluster, 1:w173:bool, 3:w170:path)  [unwired: 5 in, 1 out]
                n129 = case shown="No Error" w168 {
                  tunnel: w173 -> [w178 w195]
                  tunnel: w172 -> [w177 _]
                  tunnel: w170 -> [w175 _]
                  tunnel: w167 -> [w174 _]
                  frame No Error {
                    n130 = Strip Path(path=w175) -> (name=w176:string)  [unwired: 1 out]
                    n131 = case "Load File?" shown="False" w178 {
                      tunnel: w177 -> [w191 _]
                      tunnel: w176 -> [w185 _]
                      tunnel: w175 -> [w186 _]
                      tunnel: w174 -> [w179 _]
                      frame False {
                        n132 = call "PrepareSignals.vi"("SetValueInfo in"=w179, "setfile path"=w186, "Enum"=enum16{"Save", "Load"}."Load", "Display Message to \nUser"=TRUE ("Display Message to \nUser"), "DIMControSet in"=w191) -> ("indexed loaded Array"=w189:dbl[][], "Name Array"=w188:string[], "DIMControSet out"=w190:refnum<vi>[])  [unwired: 4 in]
                        n133 = call "CompareArrays.vi"("indexed loaded Array"=w189, "Name Array"=w188, "DIMControSet"=w190) -> ("Table for loading values"=w187:string[][])  [unwired: 4 in]
                        n134 = call "LoadSet.vi"("File Name In"=w185, "output array"=w187) -> ("File Name out"=w184:string, "Accepted"=w183:bool)  [unwired: 8 in]
                        n135 = case "Accepted?" shown="True" w183 {
                          tunnel: w184 -> [_ w194]
                          tunnel: "deceltobun" ("string") -> [_ w193]
                          frame False {
                          }
                          frame True {
                            n136 = call "UpdateLastLoadedFile.vi"("LoadOrSave"=enum16{"Load", "Save"}."Load", "GUIName"=w193, "FileNameIn"=w194) -> ()  [unwired: 13 in]
                          }
                        }
                      }
                      frame True {
                      }
                    }
                  }
                  frame Error {
                    n137 = Not(x=w195) -> (.not. x?=w196:bool)
                    n138 = call "Display Message to User"("Enable"=w196) -> ()  [unwired: 9 in, 2 out]
                  }
                }
              }
              frame "BUNAPP_FILE_ZERO" {
                w201 = "All Signals Go To Zero.set" ("File Name")
                # "Set Voltages to Zero"
                n139 = property on="SetFileLocation" class="Path"() -> ("Value"=w199:path)  [unwired: 2 in, 2 out]
                n140 = Build Path(base path=w199, name or relative path=w201) -> (appended path=w200:path)
                n141 = call "PrepareSignals.vi"("SetValueInfo in"=w197, "setfile path"=w200, "Enum"=enum16{"Save", "Load"}."Load", "Display Message to \nUser"=TRUE ("Display Message to \nUser"), "DIMControSet in"=w210) -> ("indexed loaded Array"=w208:dbl[][], "Name Array"=w207:string[], "DIMControSet out"=w209:refnum<vi>[])  [unwired: 4 in]
                n142 = call "CompareArrays.vi"("indexed loaded Array"=w208, "Name Array"=w207, "DIMControSet"=w209) -> ("Table for loading values"=w206:string[][])  [unwired: 4 in]
                n143 = call "LoadSet.vi"("File Name In"=w201, "output array"=w206) -> ("File Name out"=w204:string, "Accepted"=w205:bool)  [unwired: 8 in]
                n144 = case "Accepted?" shown="True" w205 {
                  tunnel: w204 -> [_ w213]
                  tunnel: "deceltobun" ("string") -> [_ w212]
                  frame False {
                  }
                  frame True {
                    n145 = call "UpdateLastLoadedFile.vi"("LoadOrSave"=enum16{"Load", "Save"}."Load", "GUIName"=w212, "FileNameIn"=w213) -> ()  [unwired: 13 in]
                  }
                }
              }
              frame "Legend" {
                # "Open Legend"
                n146 = call "Legend.vi"("i ref in"=refnum<vi> refnum) -> ("i ref out"=→"i ref out":refnum<vi>)  [unwired: 10 in]
              }
              frame "BUNAPP_FILE_EXIT" {
                # "Exit"
              }
            }
          }
          event Value Change {
            n147 = event-data() -> ("NewVal"=w220:T1)  [unwired: 1 in]
            n148 = stacked-sequence {
              tunnel: w220 -> [w226 _]
              tunnel: w218 -> [_ w244]
              tunnel: w217 -> [_ w238]
              frame #0 {
                # "Update Set File Location"
                n149 = Unbundle By Name(w226) -> ("data"=w231:string, "no link"=w230:bool, "quality"=w229:i32)
                n150 = case "Link?" shown="True" w230 {
                  tunnel: w229 -> [w235 _]
                  tunnel: [w234 UtilityLib.valueStatus."no info available" ("valueStatus")] -> w232
                  tunnel: w231 -> [w233 _]
                  tunnel: [w233 w236] -> w227
                  frame False {
                    n151 = call "CoreLib.quality 2 status.vi"("quality"=w235) -> ("valueStatus"=w234:T4)  [unwired: 18 in]
                  }
                  frame True {
                    n152 = call "EmptyString.vi"() -> ("String"=w236:string)
                  }
                }
                n153 = Type Cast(type="" ("regular expression"), x=w227) -> (*(type *) &x=w225:string)
                n154 = String To Path(string=w225) -> (path=w221:path)
                n155 = control-ref of="SetFileLocation"() -> (w223:refnum<vi>)
                n156 = Build Path(base path=w221, name or relative path="deceltobunControl") -> (appended path=w222:path)
                n157 = property class="Path"(reference=w223, "Value"=w222) -> ()  [unwired: 1 in, 2 out]
                n158 = call "UtilityLib.set color of GUI object.vi"("GUI object Ref"=w223, "valueStatus"=w232) -> ()  [unwired: 17 in, 1 out]
              }
              frame #1 {
                # "Update Last Loaded File"
                n159 = control-ref of="SetFileLocation"() -> (w242:refnum<vi>)
                n160 = control-ref of="Last Loaded File"() -> (w243:refnum<vi>)
                n161 = control-ref of="Last Loaded File_Data"() -> (w241:refnum<vi>)
                n162 = property class="Clust (strict)"(reference=w241) -> ("Value"=w240:T5)  [unwired: 1 in, 2 out]
                n163 = call "LastLoadedFile.vi"("SetFileLocation"=w242, "Last Loaded File"=w243, "GUIName"="deceltobun", "DIMControSet in"=w244, "SetValueInfo in"=w238, "NewVal"=w240) -> ()  [unwired: 14 in]
              }
            }
          }
          event Value Change {
            # "Update Last Loaded File"
            n164 = event-data() -> ("NewVal"=w248:T1)  [unwired: 1 in]
            n165 = control-ref of="Last Loaded File"() -> (w249:refnum<vi>)
            n166 = control-ref of="SetFileLocation"() -> (w250:refnum<vi>)
            n167 = call "LastLoadedFile.vi"("SetFileLocation"=w250, "Last Loaded File"=w249, "GUIName"="deceltobun", "DIMControSet in"=w246, "SetValueInfo in"=w245, "NewVal"=w248) -> ()  [unwired: 14 in]
          }
          event Value Change {
            # "Find Monitor Value Index"
            # "Updating a Monitor Value"
            n168 = event-data() -> ("CtlRef"=w256:refnum<vi>, "NewVal"=w259:T2)  [unwired: 1 in, 4 out]
            n169 = Search 1D Array(1D array=w257, element=w256) -> (index of element=w255:i32)  [unwired: 1 in]
            n170 = Index Array(array=w254, index=w255) -> (element=w253:refnum<vi>)
            n171 = Not A Number/Path/Refnum?(number/path/refnum=w253) -> (NaN/Path/Refnum?=w252:bool)
            n172 = case "Indicator does not exists?" shown="False" w252 {
              tunnel: w259 -> [_ w266]
              tunnel: w253 -> [_ w260]
              frame True {
              }
              frame False {
                n173 = Unbundle By Name(w266) -> ("data"=w262:dbl, "no link"=w263:bool, "quality"=w265:i32)
                n174 = case shown="False" w263 {
                  tunnel: w265 -> [w269 _]
                  tunnel: [w268 UtilityLib.valueStatus."no info available" ("valueStatus")] -> w264
                  tunnel: w262 -> [w267 _]
                  tunnel: [w267 inf] -> w261
                  frame False {
                    n175 = call "CoreLib.quality 2 status.vi"("quality"=w269) -> ("valueStatus"=w268:T4)  [unwired: 18 in]
                  }
                  frame True {
                  }
                }
                n176 = property class="DigNum (strict)"(reference=w260, "Value"=w261) -> ()  [unwired: 1 in, 2 out]
                n177 = call "TextColor.vi"("valueStatus"=w264, "reference"=w260) -> ()  [unwired: 10 in]
              }
            }
          }
          event Value Change {
            n178 = event-data() -> ("CtlRef"=w275:refnum<vi>)  [unwired: 1 in, 5 out]
            n179 = property on="FileUpToDate" class="Bool (strict)"() -> ("Value"=w272:bool)  [unwired: 2 in, 2 out]
            n180 = call "FileUpToDate.vi"("FileUpToDate in"=w272, "DIMControSet out"=w274, "CtlRef"=w275) -> ("FileUpToDate out"=w273:bool)  [unwired: 16 in]
            n181 = property on="FileUpToDate" class="Bool (strict)"("Value"=w273) -> ()  [unwired: 2 in, 2 out]
          }
          event "PreBunLens", "Decel", "DecelLens", "BOB2DefY", "BOB2DefX", "Q90CylLens", "ISDefX", "Q90BOB3Lens", "Q90DefMain", "BOB2Q90Lens", "BOB3DefX", "BOB3DefY", "Q90PlanLens", "ISDefY", "Q90PlanDefY": Value Change {
            # "Find sub-panel index"
            # "opening or closing a sub-panel"
            n182 = event-data() -> ("CtlRef"=w278:refnum<vi>)  [unwired: 1 in, 3 out]
            n183 = Search 1D Array(1D array=w277, element=w278) -> (index of element=w283:i32)  [unwired: 1 in]
            n184 = Index Array(array=w284, index=w283) -> (element=w281:refnum<vi>)
            n185 = invoke class="Bool" method="Reinit To Default"(reference=w278) -> ()  [unwired: 2 in, 3 out]
            n186 = property class="VI"(reference=w281) -> ("Front Panel.Open"=w280:bool)  [unwired: 1 in, 2 out]
            n187 = case "Panel Already Open?" shown="True" w280 {
              tunnel: w281 -> [_ w288]
              tunnel: [w286 refnum<vi> refnum ("vi reference")] -> w279
              tunnel: w278 -> [w285 _]
              frame False {
                n188 = call "OpenPanel.vi"("CtlRef"=w285) -> ("vi reference"=w286:refnum<vi>)  [unwired: 2 in]
              }
              frame True {
                n189 = call "PanelClose.vi"("vi reference"=w288) -> ()
              }
            }
            n190 = Replace Array Subset(array=w284, new element=w279, index=w283) -> (w282:refnum<vi>[])
          }
          event "Close All Panels": Value Change {
            # "Close All Panels"
            n191 = event-data() -> ()  [unwired: 1 in, 6 out]
            n192 = case "Close Open Panels?" shown="True" "Close All Panels" {
              tunnel: w291 -> [w292 w294]
              tunnel: [w292 w293] -> w289
              frame False {
              }
              frame True {
                n193 = for "Close Open Panels" {
                  tunnel: w294 -> [w296] mode=indexing
                  tunnel: w294 -> [w295]
                  tunnel: [w295] -> w293
                  n194 = call "PanelClose.vi"("vi reference"=w296) -> ()
                }
              }
            }
          }
          event "DIM Error": Value Change {
            # "DIM Error"
            n195 = event-data() -> ("NewVal"=w297:bool)  [unwired: 1 in]
            n196 = call "Display Message to User"("Enable"=w297) -> ()  [unwired: 9 in, 2 out]
          }
          event Timeout {
            # "Timeout"
            n197 = event-data() -> ()  [unwired: 1 in, 3 out]
          }
          event Panel Close? {
            n198 = event-data() -> ()  [unwired: 1 in, 4 out]
            n199 = stacked-sequence {
              tunnel: w303 -> [w310 _]
              tunnel: w302 -> [w308 _]
              tunnel: w301 -> [w307 _]
              tunnel: w300 -> [w306 _]
              frame #0 {
                # "Release DIM Services"
                n200 = for "Close Open Panels" {
                  tunnel: w310 -> [w320] mode=indexing
                  n201 = call "PanelClose.vi"("vi reference"=w320) -> ()
                }
                n202 = for "For Each Service" {
                  tunnel: w306 -> [w312] mode=indexing
                  n203 = Not A Number/Path/Refnum?(number/path/refnum=w312) -> (NaN/Path/Refnum?=w311:bool)
                  n204 = case "Not a Reference?" shown="False" w311 {
                    tunnel: w312 -> [w313 _]
                    frame False {
                      n205 = call "DimIndicators.dic_release_service.vi"("controlRef"=w313) -> ()  [unwired: 18 in, 1 out]
                    }
                    frame True {
                    }
                  }
                }
                n206 = for "For Each Service" {
                  tunnel: w307 -> [w315] mode=indexing
                  n207 = Not A Number/Path/Refnum?(number/path/refnum=w315) -> (NaN/Path/Refnum?=w314:bool)
                  n208 = case "Not a Reference?" shown="False" w314 {
                    tunnel: w315 -> [w316 _]
                    frame False {
                      n209 = call "DimIndicators.dic_release_service.vi"("controlRef"=w316) -> ()  [unwired: 18 in, 1 out]
                    }
                    frame True {
                    }
                  }
                }
                n210 = for "For Each Service" {
                  tunnel: w308 -> [w318] mode=indexing
                  n211 = Not A Number/Path/Refnum?(number/path/refnum=w318) -> (NaN/Path/Refnum?=w317:bool)
                  n212 = case "Not a Reference?" shown="False" w317 {
                    tunnel: w318 -> [w319 _]
                    frame False {
                      n213 = call "DimIndicators.dic_release_service.vi"("controlRef"=w319) -> ()  [unwired: 18 in, 1 out]
                    }
                    frame True {
                    }
                  }
                }
                n214 = control-ref of="SetFileLocation_Data"() -> (w305:refnum<vi>)
                n215 = control-ref of="Last Loaded File_Data"() -> (w309:refnum<vi>)
                n216 = call "DimIndicators.dic_release_service.vi"("controlRef"=w305) -> ()  [unwired: 18 in, 1 out]
                n217 = call "DimIndicators.dic_release_service.vi"("controlRef"=w309) -> ()  [unwired: 18 in, 1 out]
              }
              frame #1 {
                # "Close Front Panel"
                n218 = Current VI's Path() -> (path=w321:path)
                n219 = Open VI Reference(vi path=w321) -> (vi reference=w323:refnum<vi>, error out=w324:errorcluster)  [unwired: 5 in]
                n220 = property class="VI"(reference=w323, error in=w324, "Front Panel Window:Open"=FALSE) -> ()  [unwired: 2 out]
              }
            }
            n221 = event-data() -> ()  [unwired: 2 in, 1 out]
          }
        }
      }
    }
    frame #3 {
      n222 = stacked-sequence "Close Connections to DIM" {
        tunnel: w328 -> [w330 _ _]
        tunnel: w327 -> [w334 _ _]
        tunnel: w326 -> [w331 _ _]
        tunnel: w325 -> [w332 _ _]
        frame #0 {
          # "Release DIM Services"
          n223 = for "For Each Service" {
            tunnel: w332 -> [w342] mode=indexing
            n224 = Not A Number/Path/Refnum?(number/path/refnum=w342) -> (NaN/Path/Refnum?=w341:bool)
            n225 = case "Not a Reference?" shown="False" w341 {
              tunnel: w342 -> [w343 _]
              frame False {
                n226 = call "DimIndicators.dic_release_service.vi"("controlRef"=w343) -> ()  [unwired: 18 in, 1 out]
              }
              frame True {
              }
            }
          }
          n227 = for "For Each Service" {
            tunnel: w331 -> [w339] mode=indexing
            n228 = Not A Number/Path/Refnum?(number/path/refnum=w339) -> (NaN/Path/Refnum?=w338:bool)
            n229 = case "Not a Reference?" shown="False" w338 {
              tunnel: w339 -> [w340 _]
              frame False {
                n230 = call "DimIndicators.dic_release_service.vi"("controlRef"=w340) -> ()  [unwired: 18 in, 1 out]
              }
              frame True {
              }
            }
          }
          n231 = for "For Each Service" {
            tunnel: w330 -> [w336] mode=indexing
            n232 = Not A Number/Path/Refnum?(number/path/refnum=w336) -> (NaN/Path/Refnum?=w335:bool)
            n233 = case "Not a Reference?" shown="False" w335 {
              tunnel: w336 -> [w337 _]
              frame False {
                n234 = call "DimIndicators.dic_release_service.vi"("controlRef"=w337) -> ()  [unwired: 18 in, 1 out]
              }
              frame True {
              }
            }
          }
          n235 = control-ref of="Last Loaded File_Data"() -> (w333:refnum<vi>)
          n236 = control-ref of="SetFileLocation_Data"() -> (w329:refnum<vi>)
          n237 = for "Close Open Panels" {
            tunnel: w334 -> [w344] mode=indexing
            n238 = call "PanelClose.vi"("vi reference"=w344) -> ()
          }
          n239 = call "DimIndicators.dic_release_service.vi"("controlRef"=w333) -> ()  [unwired: 18 in, 1 out]
          n240 = call "DimIndicators.dic_release_service.vi"("controlRef"=w329) -> ()  [unwired: 18 in, 1 out]
        }
        frame #1 {
          # "Close Front Panel"
          n241 = Current VI's Path() -> (path=w348:path)
          n242 = Open VI Reference(vi path=w348) -> (vi reference=w346:refnum<vi>, error out=w345:errorcluster)  [unwired: 5 in]
          n243 = property class="VI"(reference=w346, error in=w345, "Front Panel Window:Open"=FALSE) -> ()  [unwired: 2 out]
        }
        frame #2 {
          # "Stop Panel"
          n244 = Stop(stop? (T)=TRUE) -> ()
        }
      }
    }
  }
  n245 = call "LVDimInterface.dim_operate.vi"("DNSNode"="lebit-balcony") -> ()  [unwired: 19 in]
  n246 = call "DIM-Error.vi"() -> ("DIM Error"=w1:bool)  [unwired: 11 in]
  n247 = property on="DIM Error" class="Bool (strict)"("Val(Sgnl)"=w1) -> ()  [unwired: 2 in, 2 out]
